vi "Toggle Continuous Output.vi"(1 "Input Boolean":bool) -> (0 "Output":bool)   [LabVIEW 2013]
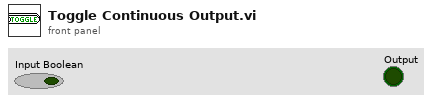
[diagram p1: front panel]
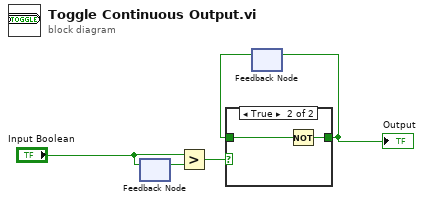
[diagram p0: block diagram]
diagram:
  n1 = feedback #1() -> (w4:bool)  [unwired: 1 in]
  n2 = feedback-in #1("Input Boolean") -> ()
  n3 = Greater?(x="Input Boolean", y=w4) -> (0:w2:bool)
  n4 = feedback #2() -> (w1:bool)  [unwired: 1 in]
  n5 = case shown="True" w2 {
    tunnel: [w6 w8] -> w5
    tunnel: w1 -> [w6 w7]
    frame False {
    }
    frame True {
      n6 = Not(x=w7) -> (.not. x?=w8:bool)
    }
  }
  "Output" <- w5
  n7 = feedback-in #2(w5) -> ()
